vi "Update Position.vi"(8 "error in (no error)":errorcluster, 10 "Diff":cluster{"x":i16, "y":i16}, 11 "Rectangle Border in":refnum<class "Rectangle Border.lvclass">) -> (0 "error out":errorcluster, 1 "EndPoint":cluster{"x":i16, "y":i16}, 2 "StartPoint":cluster{"x":i16, "y":i16}, 3 "Rectangle Border out":refnum<class "Rectangle Border.lvclass">)   [LabVIEW 2015, in "Rectangle Border.lvclass"]
uses:
  Rectangle Border.lvclass
  Scalable Border/Scalable Border.lvclass/Scalable Border.ctl
  Rectangle Border.lvclass/Rectangle Border.ctl
  Scalable Border/Scalable Border.lvclass
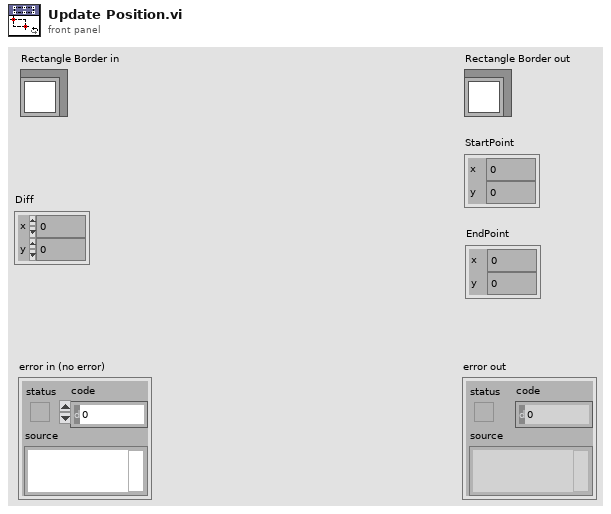
[diagram p1: front panel]
types:
  T1 = cluster{"left":i16, "top":i16, "right":i16, "bottom":i16}
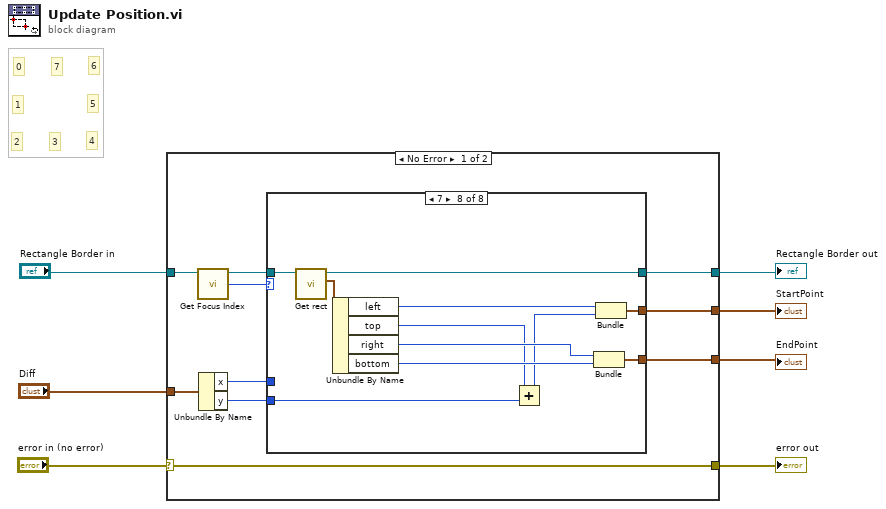
[diagram p0: block diagram]
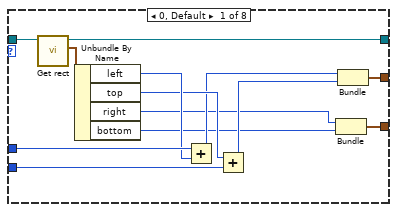
[diagram p2: hidden frame]
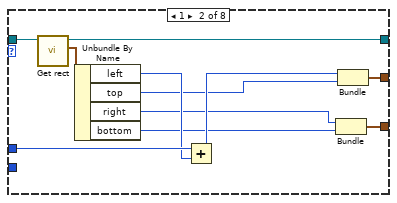
[diagram p3: hidden frame]
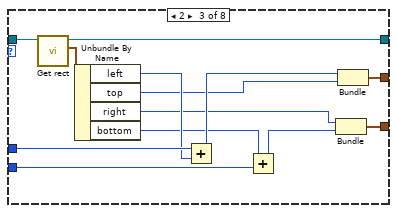
[diagram p4: hidden frame]
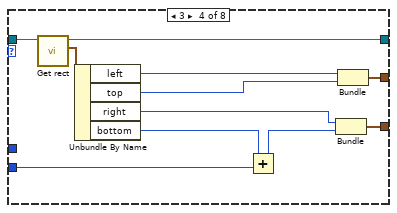
[diagram p5: hidden frame]
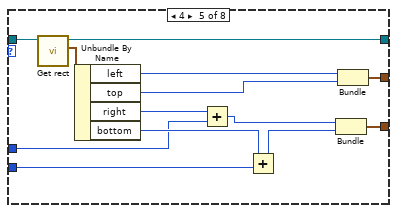
[diagram p6: hidden frame]
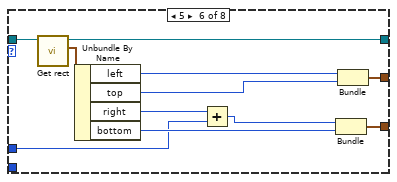
[diagram p7: hidden frame]
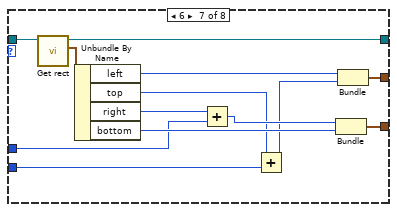
[diagram p8: hidden frame]
diagram:
  # "4"
  # "5"
  # "6"
  # "3"
  # "7"
  # "2"
  # "1"
  # "0"
  n1 = case shown="No Error" "error in (no error)" {
    selector: "error in (no error)" -> [w17 w115]
    tunnel: [w10 w114] -> w3
    tunnel: "Diff" -> [w13 _]
    tunnel: [w17 w115] -> w5
    tunnel: "Rectangle Border in" -> [w14 w114]
    tunnel: [w9 _] -> w2
    tunnel: [w8 _] -> w1
    frame No Error {
      n2 = call "Get Focus Index.vi"("Scalable Border in"=w14) -> ("Focus Index"=w16:i8, "Scalable Border out"=w15:refnum<class "Rectangle Border.lvclass">)  [unwired: 8 in, 1 out]
      n3 = Unbundle By Name(w13) -> ("x"=w12:i16, "y"=w11:i16)
      n4 = case shown="7" w16 {
        tunnel: w15 -> [w30 w41 w54 w65 w78 w89 w102 w113]
        tunnel: w12 -> [w29 w40 w53 _ w68 w81 w96 _]
        tunnel: w11 -> [w27 _ w43 w57 w71 _ w93 w107]
        tunnel: [w25 w38 w51 w64 w77 w88 w101 w112] -> w10
        tunnel: [w19 w33 w47 w61 w75 w86 w99 w110] -> w9
        tunnel: [w18 w32 w46 w60 w74 w85 w98 w109] -> w8
        frame 0, Default {
          n5 = call "Get rect.vi"("Rectangle Border in"=w30) -> ("rect"=w24:T1, "Rectangle Border out"=w25:refnum<class "Rectangle Border.lvclass">)  [unwired: 8 in, 1 out]
          n6 = Unbundle By Name(w24) -> ("left"=w28:i16, "top"=w26:i16, "right"=w21:i16, "bottom"=w20:i16)
          n7 = Add(x=w29, y=w28) -> (x+y=w23:i16)
          n8 = Add(x=w26, y=w27) -> (x+y=w22:i16)
          n9 = Bundle("right"=w21, "bottom"=w20) -> (w18:cluster{"right":i16, "bottom":i16})  [unwired: 1 in]
          n10 = Bundle(w23, w22) -> (w19:cluster{i16, i16})  [unwired: 1 in]
        }
        frame 1 {
          n11 = call "Get rect.vi"("Rectangle Border in"=w41) -> ("rect"=w37:T1, "Rectangle Border out"=w38:refnum<class "Rectangle Border.lvclass">)  [unwired: 8 in, 1 out]
          n12 = Unbundle By Name(w37) -> ("left"=w39:i16, "top"=w31:i16, "right"=w35:i16, "bottom"=w34:i16)
          n13 = Add(x=w40, y=w39) -> (x+y=w36:i16)
          n14 = Bundle("right"=w35, "bottom"=w34) -> (w32:cluster{"right":i16, "bottom":i16})  [unwired: 1 in]
          n15 = Bundle(w36, "top"=w31) -> (w33:cluster{i16, "top":i16})  [unwired: 1 in]
        }
        frame 2 {
          n16 = call "Get rect.vi"("Rectangle Border in"=w54) -> ("rect"=w50:T1, "Rectangle Border out"=w51:refnum<class "Rectangle Border.lvclass">)  [unwired: 8 in, 1 out]
          n17 = Unbundle By Name(w50) -> ("left"=w52:i16, "top"=w45:i16, "right"=w48:i16, "bottom"=w44:i16)
          n18 = Add(x=w53, y=w52) -> (x+y=w49:i16)
          n19 = Add(x=w44, y=w43) -> (x+y=w42:i16)
          n20 = Bundle("right"=w48, w42) -> (w46:cluster{"right":i16, i16})  [unwired: 1 in]
          n21 = Bundle(w49, "top"=w45) -> (w47:cluster{i16, "top":i16})  [unwired: 1 in]
        }
        frame 3 {
          n22 = call "Get rect.vi"("Rectangle Border in"=w65) -> ("rect"=w63:T1, "Rectangle Border out"=w64:refnum<class "Rectangle Border.lvclass">)  [unwired: 8 in, 1 out]
          n23 = Unbundle By Name(w63) -> ("left"=w55:i16, "top"=w59:i16, "right"=w62:i16, "bottom"=w58:i16)
          n24 = Add(x=w58, y=w57) -> (x+y=w56:i16)
          n25 = Bundle("right"=w62, w56) -> (w60:cluster{"right":i16, i16})  [unwired: 1 in]
          n26 = Bundle("left"=w55, "top"=w59) -> (w61:cluster{"left":i16, "top":i16})  [unwired: 1 in]
        }
        frame 4 {
          n27 = call "Get rect.vi"("Rectangle Border in"=w78) -> ("rect"=w76:T1, "Rectangle Border out"=w77:refnum<class "Rectangle Border.lvclass">)  [unwired: 8 in, 1 out]
          n28 = Unbundle By Name(w76) -> ("left"=w69:i16, "top"=w73:i16, "right"=w67:i16, "bottom"=w72:i16)
          n29 = Add(x=w67, y=w68) -> (x+y=w66:i16)
          n30 = Add(x=w72, y=w71) -> (x+y=w70:i16)
          n31 = Bundle(w66, w70) -> (w74:cluster{i16, i16})  [unwired: 1 in]
          n32 = Bundle("left"=w69, "top"=w73) -> (w75:cluster{"left":i16, "top":i16})  [unwired: 1 in]
        }
        frame 5 {
          n33 = call "Get rect.vi"("Rectangle Border in"=w89) -> ("rect"=w87:T1, "Rectangle Border out"=w88:refnum<class "Rectangle Border.lvclass">)  [unwired: 8 in, 1 out]
          n34 = Unbundle By Name(w87) -> ("left"=w82:i16, "top"=w84:i16, "right"=w80:i16, "bottom"=w83:i16)
          n35 = Add(x=w80, y=w81) -> (x+y=w79:i16)
          n36 = Bundle(w79, "bottom"=w83) -> (w85:cluster{i16, "bottom":i16})  [unwired: 1 in]
          n37 = Bundle("left"=w82, "top"=w84) -> (w86:cluster{"left":i16, "top":i16})  [unwired: 1 in]
        }
        frame 6 {
          n38 = call "Get rect.vi"("Rectangle Border in"=w102) -> ("rect"=w100:T1, "Rectangle Border out"=w101:refnum<class "Rectangle Border.lvclass">)  [unwired: 8 in, 1 out]
          n39 = Unbundle By Name(w100) -> ("left"=w91:i16, "top"=w92:i16, "right"=w95:i16, "bottom"=w97:i16)
          n40 = Add(x=w95, y=w96) -> (x+y=w94:i16)
          n41 = Add(x=w92, y=w93) -> (x+y=w90:i16)
          n42 = Bundle(w94, "bottom"=w97) -> (w98:cluster{i16, "bottom":i16})  [unwired: 1 in]
          n43 = Bundle("left"=w91, w90) -> (w99:cluster{"left":i16, i16})  [unwired: 1 in]
        }
        frame 7 {
          n44 = call "Get rect.vi"("Rectangle Border in"=w113) -> ("rect"=w111:T1, "Rectangle Border out"=w112:refnum<class "Rectangle Border.lvclass">)  [unwired: 8 in, 1 out]
          n45 = Unbundle By Name(w111) -> ("left"=w103:i16, "top"=w105:i16, "right"=w106:i16, "bottom"=w108:i16)
          n46 = Add(x=w105, y=w107) -> (x+y=w104:i16)
          n47 = Bundle("right"=w106, "bottom"=w108) -> (w109:cluster{"right":i16, "bottom":i16})  [unwired: 1 in]
          n48 = Bundle("left"=w103, w104) -> (w110:cluster{"left":i16, i16})  [unwired: 1 in]
        }
      }
    }
    frame Error {
    }
  }
  "error out" <- w5
  "Rectangle Border out" <- w3
  "EndPoint" <- w1
  "StartPoint" <- w2
